vi "Get Property.vi"(10 "Ctl Ref":refnum<vi>, 11 "FontUIP In":refnum<class "FontUIP.lvclass">) -> (0 "Error Out":errorcluster, 3 "FontUIP Out":refnum<class "FontUIP.lvclass">)   [LabVIEW 2016, in "FontUIP.lvclass"]
doc: "Overwrite this abstract method to implement child behavior for getting the property from the VI Server Control and into the UIP private data."
uses:
  FontUIP.lvclass
  FontUIP.lvclass/FontUIP.ctl
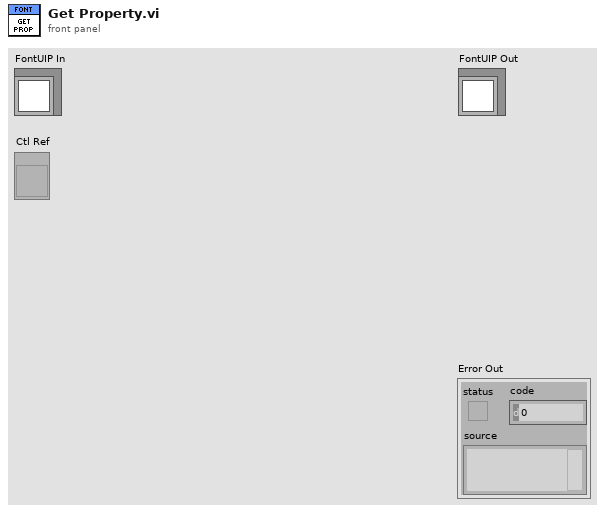
[diagram p1: front panel]
types:
  T1 = typedef "LVFontTypeDef.ctl" = cluster{"Font Name":string, "Size":u16, "Bold":bool, "Italic":bool, "Underline":bool, "Strikeout":bool, "Color":u32}
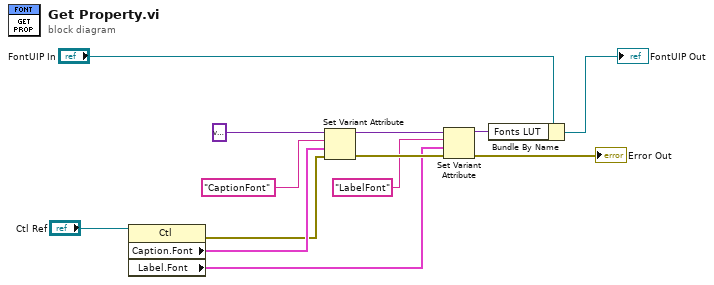
[diagram p0: block diagram]
diagram:
  n1 = property class="Ctl"(reference="Ctl Ref") -> (error out=w8:errorcluster, "Caption.Font"=w9:T1, "Label.Font"=w3:T1)  [unwired: 1 in, 1 out]
  n2 = Set Variant Attribute(Variant=variant ("variant"), name="CaptionFont", value=w9, error in=w8) -> (Variant out=w5:variant, error out=w6:errorcluster)  [unwired: 1 out]
  n3 = Set Variant Attribute(Variant=w5, name="LabelFont", value=w3, error in=w6) -> (Variant out=w2:variant, error out=→"Error Out":errorcluster)  [unwired: 1 out]
  n4 = Bundle By Name(cluster="FontUIP In", "Fonts LUT"=w2) -> (→"FontUIP Out":refnum<class "FontUIP.lvclass">)
